vi "configureTSstepProperties.vi"(8 "error in":errorcluster, 9 "PostExpression":string, 10 "Precondition":string, 11 "NewStep (in)":refnum<k7>) -> (0 "error out":errorcluster, 3 "NewStep (out)":refnum<k7>)   [LabVIEW 2010]
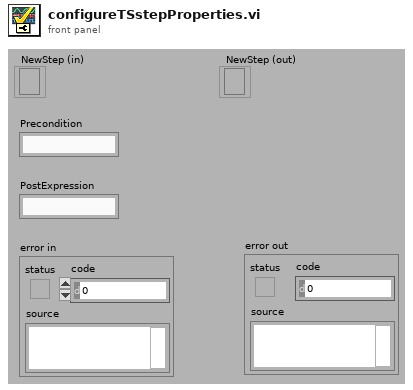
[diagram p1: front panel]
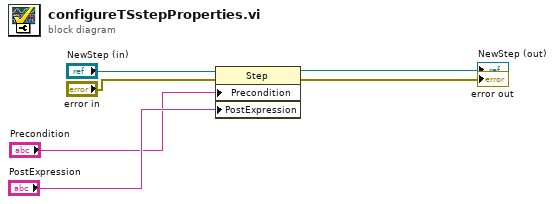
[diagram p0: block diagram]
diagram:
  n1 = property class="Step"(reference="NewStep (in)", error in="error in", "Precondition"="Precondition", "PostExpression"="PostExpression") -> (reference out=→"NewStep (out)":refnum<k7>, error out=→"error out":errorcluster)
